vi "WritebyRefNumArrV2.vi"(8 "error in":errorcluster caption="entrée d'erreur", 10 "Tableau":dbl[](array[numeric]), 11 "Ctrl Ref":refnum<vi>[](array[refnum])) -> (0 "error out":errorcluster caption="sortie d'erreur")   [LabVIEW 2019]
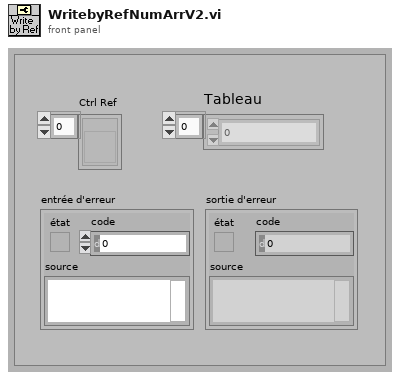
[diagram p1: front panel]
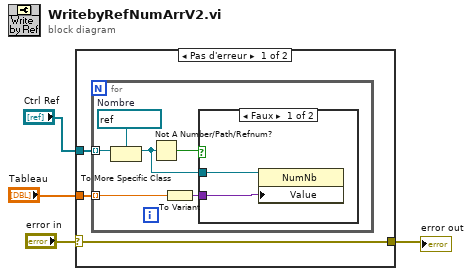
[diagram p0: block diagram]
diagram:
  n1 = case shown="Pas d'erreur" "error in" {
    selector: "error in" -> [w5 w16]
    tunnel: "Ctrl Ref" -> [w7 _]
    tunnel: "Tableau" -> [w6 _]
    tunnel: [w5 w16] -> w3
    frame No Error {
      n2 = for {
        tunnel: w7 -> [w12] mode=indexing
        tunnel: w6 -> [w11] mode=indexing
        w9 = refnum<vi> refnum  # Nombre
        n3 = To More Specific Class(target class=w9, reference=w12) -> (specific class reference=w10:refnum<vi>)  [unwired: 1 in, 1 out]
        n4 = Not A Number/Path/Refnum?(number/path/refnum=w10) -> (NaN/Path/Refnum?=w13:bool)
        n5 = To Variant(anything=w11) -> (Variant=w8:variant)
        n6 = case shown="Faux" w13 {
          tunnel: w10 -> [w15 _]
          tunnel: w8 -> [w14 _]
          frame False {
            n7 = property class="NumNb"(reference=w15, "Value"=w14) -> ()  [unwired: 1 in, 2 out]
          }
          frame True {
          }
        }
      }
    }
    frame Error {
    }
  }
  "error out" <- w3
